vi "channeldata_continued.vi"() -> ()   [LabVIEW 2019]
panel:
  out "Error Out":errorcluster
  in  "TDMS File":path=path "C:/Python/projects/nitdms/tests/tdms_files/channeldata_continued.tdms"
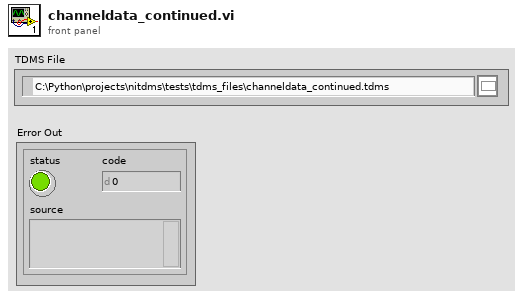
[diagram p1: front panel]
types:
  T1 = enum16{"open", "open or create", "create or replace", "create", "open (read-only)"}
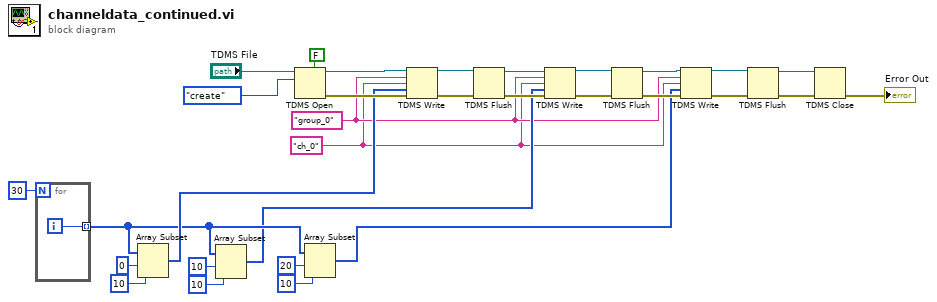
[diagram p0: block diagram]
diagram:
  w2 = "ch_0"
  w3 = "group_0"
  n1 = for {
    N: 30 -> [_]
    tunnel: [w32] -> w17 mode=indexing
    i -> [w32]
  }
  n2 = Array Subset(array=w17, index=0, length=10) -> (w20:i32[])
  n3 = Array Subset(array=w17, index=10, length=10) -> (w10:i32[])
  n4 = TDMS Open(5:FALSE ("create index file? (T)"), 10:T1."create" ("operation (0:open)"), 11:"TDMS File") -> (0:w27:errorcluster, 3:w26:refnum<k34>)  [unwired: 4 in]
  n5 = Array Subset(array=w17, index=20, length=10) -> (w1:i32[])
  n6 = TDMS Write(0:w26, 5:w3, 7:w2, 9:w20, 11:w27) -> (4:w15:refnum<k34>, 15:w16:errorcluster)  [unwired: 1 in, 2 out]
  n7 = TDMS Flush(4:w16, 7:w15) -> (0:w12:errorcluster, 3:w11:refnum<k34>)
  n8 = TDMS Write(0:w11, 5:w3, 7:w2, 9:w10, 11:w12) -> (4:w14:refnum<k34>, 15:w13:errorcluster)  [unwired: 1 in, 2 out]
  n9 = TDMS Flush(4:w13, 7:w14) -> (0:w7:errorcluster, 3:w6:refnum<k34>)
  n10 = TDMS Write(0:w6, 5:w3, 7:w2, 9:w1, 11:w7) -> (4:w8:refnum<k34>, 15:w9:errorcluster)  [unwired: 1 in, 2 out]
  n11 = TDMS Flush(4:w9, 7:w8) -> (0:w5:errorcluster, 3:w4:refnum<k34>)
  n12 = TDMS Close(8:w5, 11:w4) -> (0:→"Error Out":errorcluster)  [unwired: 1 out]
